vi "Keep Alive Test.vi"() -> ()   [LabVIEW 2020, in "Tests.lvlib"]
uses:
  Tests.lvlib
  HTTP Server/Trace Log.ctl
  HTTP Server/Trace Item.ctl
  HTTP Server/Processing Step.ctl
  <vilib>/IlluminatedG/IG HTTP Utils/HTTP Utils/Method.ctl
  KeepAliveTestController/KeepAliveTestController.lvclass
  C:/dev/lv/2020/lv-http-server/HTTP Server/Handler/Handler.lvclass
  HTTP Server/StandardFileServe/StandardFileServe.lvclass
  HTTP Server/Server/Add Connection Handler.vi
  HTTP Server/Server/Add Request Handler.vi
  HTTP Server/Server/Add Route Handler.vi
  HTTP Server/Server/Add Controller Handler.vi
  HTTP Server/Server/Add Controller.vi
  HTTP Server/Server/Add Response Handler.vi
  HTTP Server/Server/Add Complete Handler.vi
  HTTP Server/Server/Add Exception Handler.vi
  HTTP Server/Connection Handler/Connection Handler.lvclass
  HTTP Server/Request Handler/Request Handler.lvclass
  HTTP Server/Route Handler/Route Handler.lvclass
  HTTP Server/Controller Handler/Controller Handler.lvclass
  HTTP Server/Controller/Controller.lvclass
  HTTP Server/Response Handler/Response Handler.lvclass
  HTTP Server/Complete Handler/Complete Handler.lvclass
  HTTP Server/Exception Handler/Exception Handler.lvclass
  HTTP Server/Handler/Handler.lvclass
  HTTP Server/Server/Server.lvclass
  HTTP Server/RequestTraceLog/RequestTraceLog.lvclass
  HTTP Server/HTTP Server.lvlib
  <vilib>/IlluminatedG/IG HTTP Utils/HTTP Utils/HTTP Utils.lvlib
panel:
  out "Traces":T1[](array[typedef]) {"Sending" format="%_6f"; "Expires" format="%<%X %x>T"; "Created" format="%<%X %x>T"; "Waiting" format="%_6f"; "Parsing" format="%_6f"; "Processing" format="%_6f"; "Items"."Time" format="%.6f"; "Items"."Duration" format="%.6f"}
  in  "Refresh Traces":bool
  # "Request"
  # "Response"
  # "Session"
  # "Auth"
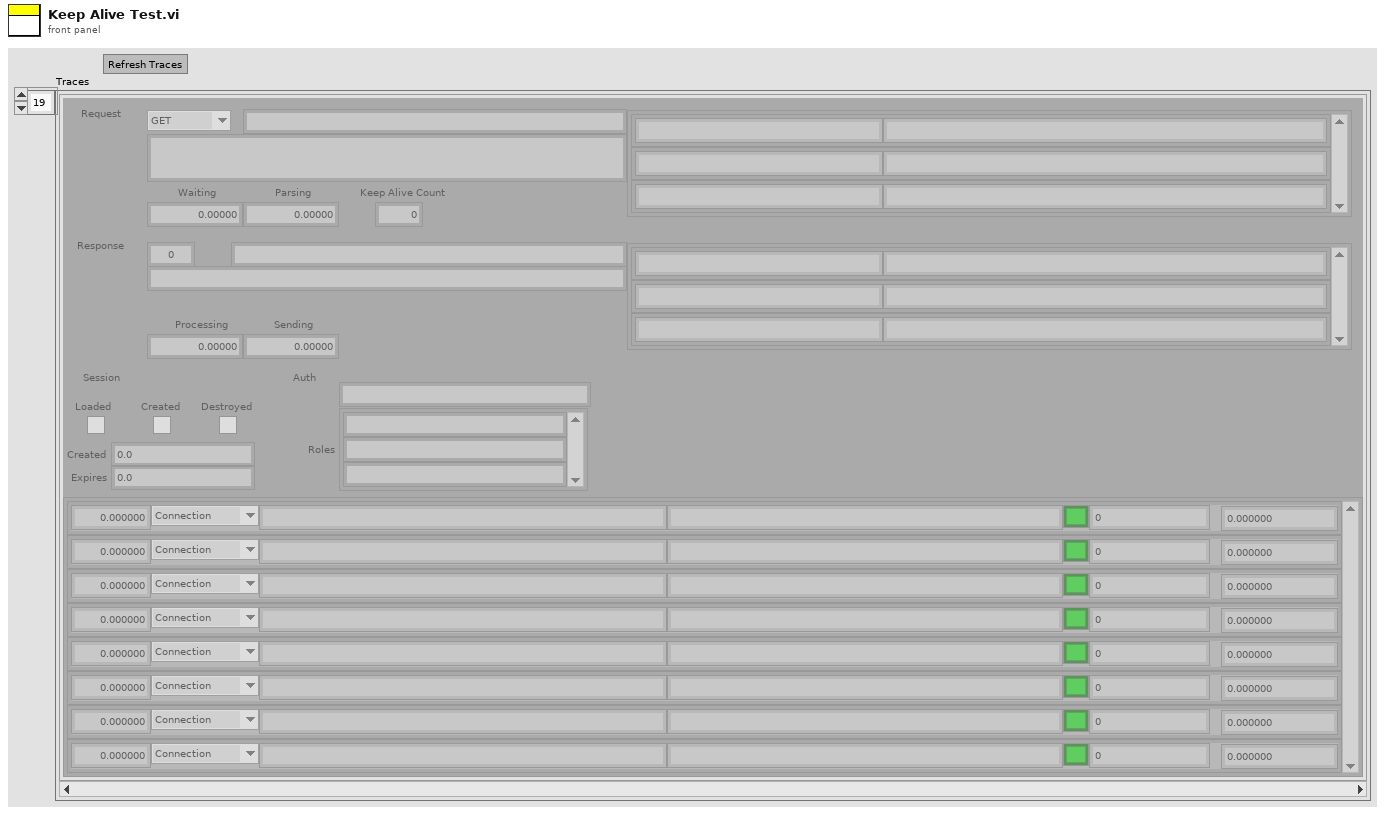
[diagram p1: front panel]
types:
  T1 = typedef "HTTP Server.lvlib/Trace Log.ctl" = cluster{"Items":T2[], "Client":string, "Target":string, "Response Type":string, "Processing":dbl, "Status":u16, "Method":T4, "Content Type":string, "Request Headers":cluster{"Name":string, "Value":string}[], "Parsing":dbl, "Waiting":dbl, "Identity":string, "Loaded":bool, "Created":bool, "Destroyed":bool, "Response Headers":cluster{"Name":string, "Value":string}[], "Created":dbl, "Expires":dbl, "Roles":string[], "Sending":dbl, "Keep Alive Count":i32}
  T2 = typedef "HTTP Server.lvlib/Trace Item.ctl" = cluster{"Duration":dbl, "Step":T3, "Class":string, "Info":string, "Status":bool, "Code":i32, "Time":dbl}
  T3 = typedef "HTTP Server.lvlib/Processing Step.ctl" = enum16{"Connection", "Request", "Routing", "Controller Init", "Controller", "Response", "Complete", "Exception"}
  T4 = typedef "HTTP Utils.lvlib/Method.ctl" = enum16{"GET", "HEAD", "POST", "PUT", "DELETE", "CONNECT", "OPTIONS", "TRACE", "PATCH"}
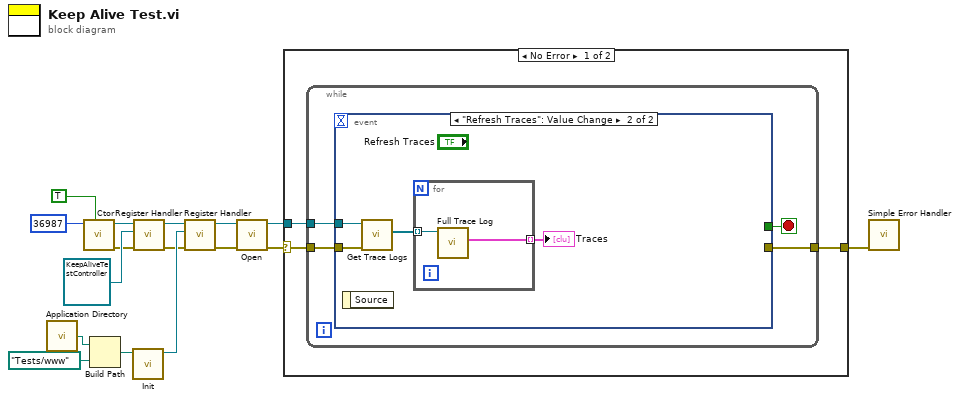
[diagram p0: block diagram]
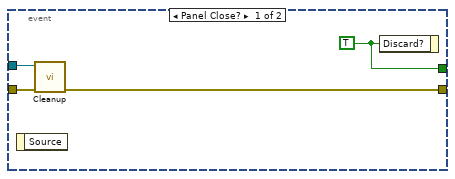
[diagram p2: hidden frame]
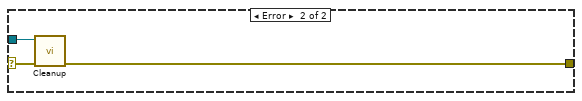
[diagram p3: hidden frame]
diagram:
  n1 = call <vilib>:"Application Directory.vi"() -> ("Application Directory"=w12:path)
  n2 = call "Ctor.vi"("Debug (F)"=TRUE, "HTTP Port (80)"=u16 36987) -> ("error out"=w6:errorcluster, "Server out"=w14:refnum<class "Server.lvclass">)  [unwired: 8 in]
  n3 = Build Path(base path=w12, name or relative path=path "Tests/www") -> (appended path=w10:path)
  n4 = call "Init.vi"("Public Root"=w10) -> ("StandardFileServe out"=w8:refnum<class "StandardFileServe.lvclass">)  [unwired: 9 in, 1 out]
  n5 = call "Register Handler.vi"("error in (no error)"=w6, "Handler"=refnum<class "KeepAliveTestController.lvclass"> refnum ("Tests.lvlib:KeepAliveTestController.lvclass"), "Server in"=w14) -> ("error out"=w5:errorcluster, "Server out"=w9:refnum<class "Server.lvclass">)  [unwired: 7 in]
  n6 = call "Register Handler.vi"("error in (no error)"=w5, "Handler"=w8, "Server in"=w9) -> ("error out"=w4:errorcluster, "Server out"=w7:refnum<class "Server.lvclass">)  [unwired: 7 in]
  n7 = call "Open.vi"("error in (no error)"=w4, "Server in"=w7) -> ("error out"=w2:errorcluster, "Server out"=w3:refnum<class "Server.lvclass">)  [unwired: 8 in]
  n8 = case shown="No Error" w2 {
    selector: w2 -> [w18 w35]
    tunnel: w3 -> [w19 w36]
    tunnel: [w17 w34] -> w1
    frame No Error {
      n9 = while {
        tunnel: w18 -> [w21]
        tunnel: w19 -> [w22]
        tunnel: [w20] -> w17
        stop <- w23 stop-if-true
        n10 = event shown="[1] \"Refresh Traces\": Value Change" {
          selector: _ -> [_ _]
          dyn-events: _ -> [_ _]
          timeout: _ -> [_ _]
          tunnel: [w27 _] -> w23
          tunnel: w22 -> [w26 w31]
          tunnel: w21 -> [w25 w30]
          tunnel: [w24 _] -> w20
          event Panel Close? {
            w27 = TRUE ("Discard?")
            n11 = event-data() -> ()  [unwired: 1 in, 1 out]
            n12 = call "Cleanup.vi"("error in (no error)"=w25, "Server in"=w26) -> ("error out"=w24:errorcluster)  [unwired: 9 in]
            n13 = event-data("Discard?"=w27) -> ()  [unwired: 1 in, 1 out]
          }
          event "Refresh Traces": Value Change {
            n14 = event-data() -> ()  [unwired: 1 in, 1 out]
            n15 = call "Get Trace Logs.vi"("error in (no error)"=w30, "Server in"=w31) -> ("Trace Logs"=w29:refnum<class "RequestTraceLog.lvclass">[])  [unwired: 7 in, 2 out]
            n16 = for {
              tunnel: w29 -> [w33] mode=indexing
              tunnel: [w32] -> w28 mode=indexing
              n17 = call "Full Trace Log.vi"("RequestTraceLog in"=w33) -> ("Trace Log"=w32:T1)  [unwired: 8 in, 2 out]
            }
            "Traces" <- w28
          }
        }
      }
    }
    frame Error {
      n18 = call "Cleanup.vi"("error in (no error)"=w35, "Server in"=w36) -> ("error out"=w34:errorcluster)  [unwired: 9 in]
    }
  }
  n19 = call <vilib>:"Simple Error Handler.vi"("error in (no error)"=w1) -> ()  [unwired: 4 in, 5 out]
